vi "Word Easy Graph.vi"(0 "report in":refnum<class "NI_report.lvclass">, 1 "graph type (col clustered)":T1(ring)=enum."xlConeColStacked100", 5 "row headers":string[](array[string]), 7 "column headers":string[](array[string]), 9 "data":dbl[][](array[numeric]) format="%.2f", 11 "error in (no error)":errorcluster, 12 "graph title (\"\")":string) -> (4 "report out":refnum<class "NI_report.lvclass">, 15 "error out":errorcluster)   [LabVIEW 2010, in "NI_ReportGenerationToolkit.lvlib"]
doc: "Inserts a graph into a Microsoft Word report."
uses:
  <vilib>/addons/_office/NI_ReportGenerationToolkit.lvlib
  <vilib>/Utility/NIReport.llb/NI_report.lvclass
  <vilib>/Utility/NIReport.llb/Word/NI_Word.lvclass
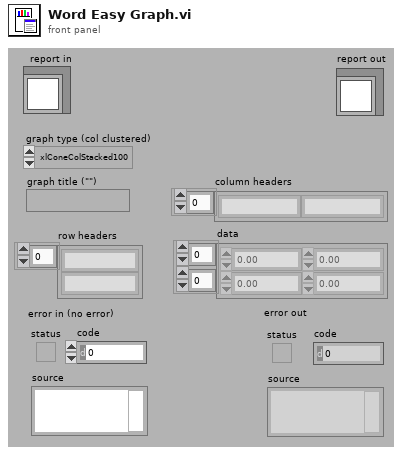
[diagram p1: front panel]
types:
  T1 = enum16{"xlColumnClustered", "xlColumnStacked", "xlColumnStacked100", "xl3DColumnClustered", "xl3DColumnStacked", "xl3DColumnStacked100", "xlBarClustered", "xlBarStacked", "xlBarStacked100", "xl3DBarClustered", "xl3DBarStacked", "xl3DBarStacked100", "xlLineStacked", "xlLineStacked100", "xlLineMarkers", "xlLineMarkersStacked", "xlLineMarkersStacked100", "xlPieOfPie", "xlPieExploded", "xl3DPieExploded", "xlBarOfPie", "xlXYScatterSmooth", "xlXYScatterSmoothNoMarkers", "xlXYScatterLines", "xlXYScatterLinesNoMarkers", "xlAreaStacked", "xlAreaStacked100", "xl3DAreaStacked", "xl3DAreaStacked100", "xlDoughnutExploded", "xlRadarMarkers", "xlRadarFilled", "xlSurface", "xlSurfaceWireframe", "xlSurfaceTopView", "xlSurfaceTopViewWireframe", "xlBubble", "xlBubble3DEffect", "xlStockHLC", "xlStockOHLC", "xlStockVHLC", "xlStockVOHLC", "xlCylinderColClustered", "xlCylinderColStacked", "xlCylinderColStacked100", "xlCylinderBarClustered", "xlCylinderBarStacked", "xlCylinderBarStacked100", "xlCylinderCol", "xlConeColClustered", "xlConeColStacked", "xlConeColStacked100", "xlConeBarClustered", "xlConeBarStacked", "xlConeBarStacked100", "xlConeCol", "xlPyramidColClustered", "xlPyramidColStacked", "xlPyramidColStacked100", "xlPyramidBarClustered", "xlPyramidBarStacked", "xlPyramidBarStacked100", "xlPyramidCol", "xl3DColumn", "xlLine", "xl3DLine", "xl3DPie", "xlPie", "xlXYScatter", "xl3DArea", "xlArea", "xlDoughnut", "xlRadar"}
  T2 = cluster{"Alignment":enum16{"Left", "Centered", "Right", "Justify"}, "Left":dbl, "Right":dbl, "Special":enum16{"(none)", "First line", "Hanging"}, "By":dbl, "Before":dbl, "After":dbl, "Line spacing":enum16{"Single", "1,5 lines", "Double", "At least", "Exactly", "Multiple"}, "At":dbl}
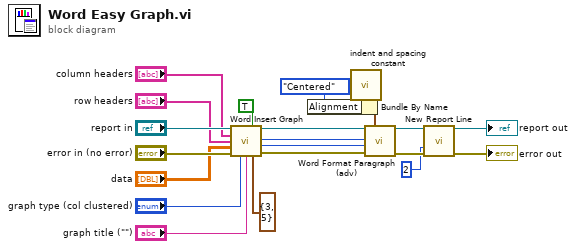
[diagram p0: block diagram]
diagram:
  n1 = call <vilib>:"Word Insert Graph.vi"("report in"="report in", "has legend? (F)"=TRUE ("has legend?"), "column headers"="column headers", "row headers"="row headers", "data"="data", "error in (no error)"="error in (no error)", "graph type (col clustered)"="graph type (col clustered)", "graph title (\"\")"="graph title (\"\")", "graph size (5, 5)"=cluster{"Height":i32, "Width":i32} {"Height"=3, "Width"=5} ("chart size")) -> ("report out"=w10:refnum<class "NI_report.lvclass">, "start"=w9:i32, "end"=w8:i32, "error out"=w11:errorcluster)  [unwired: 1 in, 2 out]
  n2 = call <vilib>:"indent and spacing constant.vi"() -> ("indent and spacing"=w12:T2)
  n3 = Bundle By Name(cluster=w12, "Alignment"=enum16{"Left", "Centered", "Right", "Justify"}."Centered") -> (w13:T2)
  n4 = call <vilib>:"Word Format Paragraph (adv).vi"("report in"=w10, "indent and spacing"=w13, "start (-1)"=w9, "end (-1)"=w8, "error in (no error)"=w11) -> ("report out"=w4:refnum<class "NI_report.lvclass">, "error out"=w5:errorcluster)  [unwired: 2 in, 7 out]
  n5 = call-dynamic "New Report Line.vi"("report in"=w4, "number of lines (1)"=2 ("number of lines"), "error in (no error)"=w5) -> ("report out"=→"report out":refnum<class "NI_report.lvclass">, "error out"=→"error out":errorcluster)  [unwired: 11 in]
